vi "mediaIntesecaoCameras_v2.vi"(9 "Lado":enum16{"Esquerdo", "Direito"}(ring) caption="Enum", 10 "Field Geometry In":T3, 11 "Cameras Array":T4[](array[typedef]) {"robots_blue"."height" format="%+4.3f"; "robots_blue"."pixel_y" format="%+4.3f"; "robots_blue"."pixel_x" format="%+4.3f"; "robots_blue"."orientation" format="%+4.3f"; "robots_blue"."y" format="%+4.3f"; "robots_blue"."confidence" format="%4.3f"; "robots_blue"."x" format="%+4.3f"; "robots_yellow"."height" format="%+4.3f"; "robots_yellow"."pixel_y" format="%+4.3f"; "robots_yellow"."pixel_x" format="%+4.3f"; "robots_yellow"."orientation" format="%+4.3f"; "robots_yellow"."y" format="%+4.3f"; "robots_yellow"."confidence" format="%4.3f"; "robots_yellow"."x" format="%+4.3f"}) -> (3 "frame out":T4 {"robots_blue"."height" format="%+4.3f"; "robots_blue"."pixel_y" format="%+4.3f"; "robots_blue"."pixel_x" format="%+4.3f"; "robots_blue"."orientation" format="%+4.3f"; "robots_blue"."y" format="%+4.3f"; "robots_blue"."confidence" format="%4.3f"; "robots_blue"."x" format="%+4.3f"; "robots_yellow"."height" format="%+4.3f"; "robots_yellow"."pixel_y" format="%+4.3f"; "robots_yellow"."pixel_x" format="%+4.3f"; "robots_yellow"."orientation" format="%+4.3f"; "robots_yellow"."y" format="%+4.3f"; "robots_yellow"."confidence" format="%4.3f"; "robots_yellow"."x" format="%+4.3f"})   [LabVIEW 2018]
uses:
  SSL Detection Frame.ctl
  SSL Detection Robot.ctl
  <vilib>/Analysis/Matrix/Datatypes/RealMatrix.ctl
  SSL Detection Ball.ctl
  <vilib>/Analysis/Matrix/NI_Matrix.lvlib
panel:
  in  "Array":T1[](array[typedef])
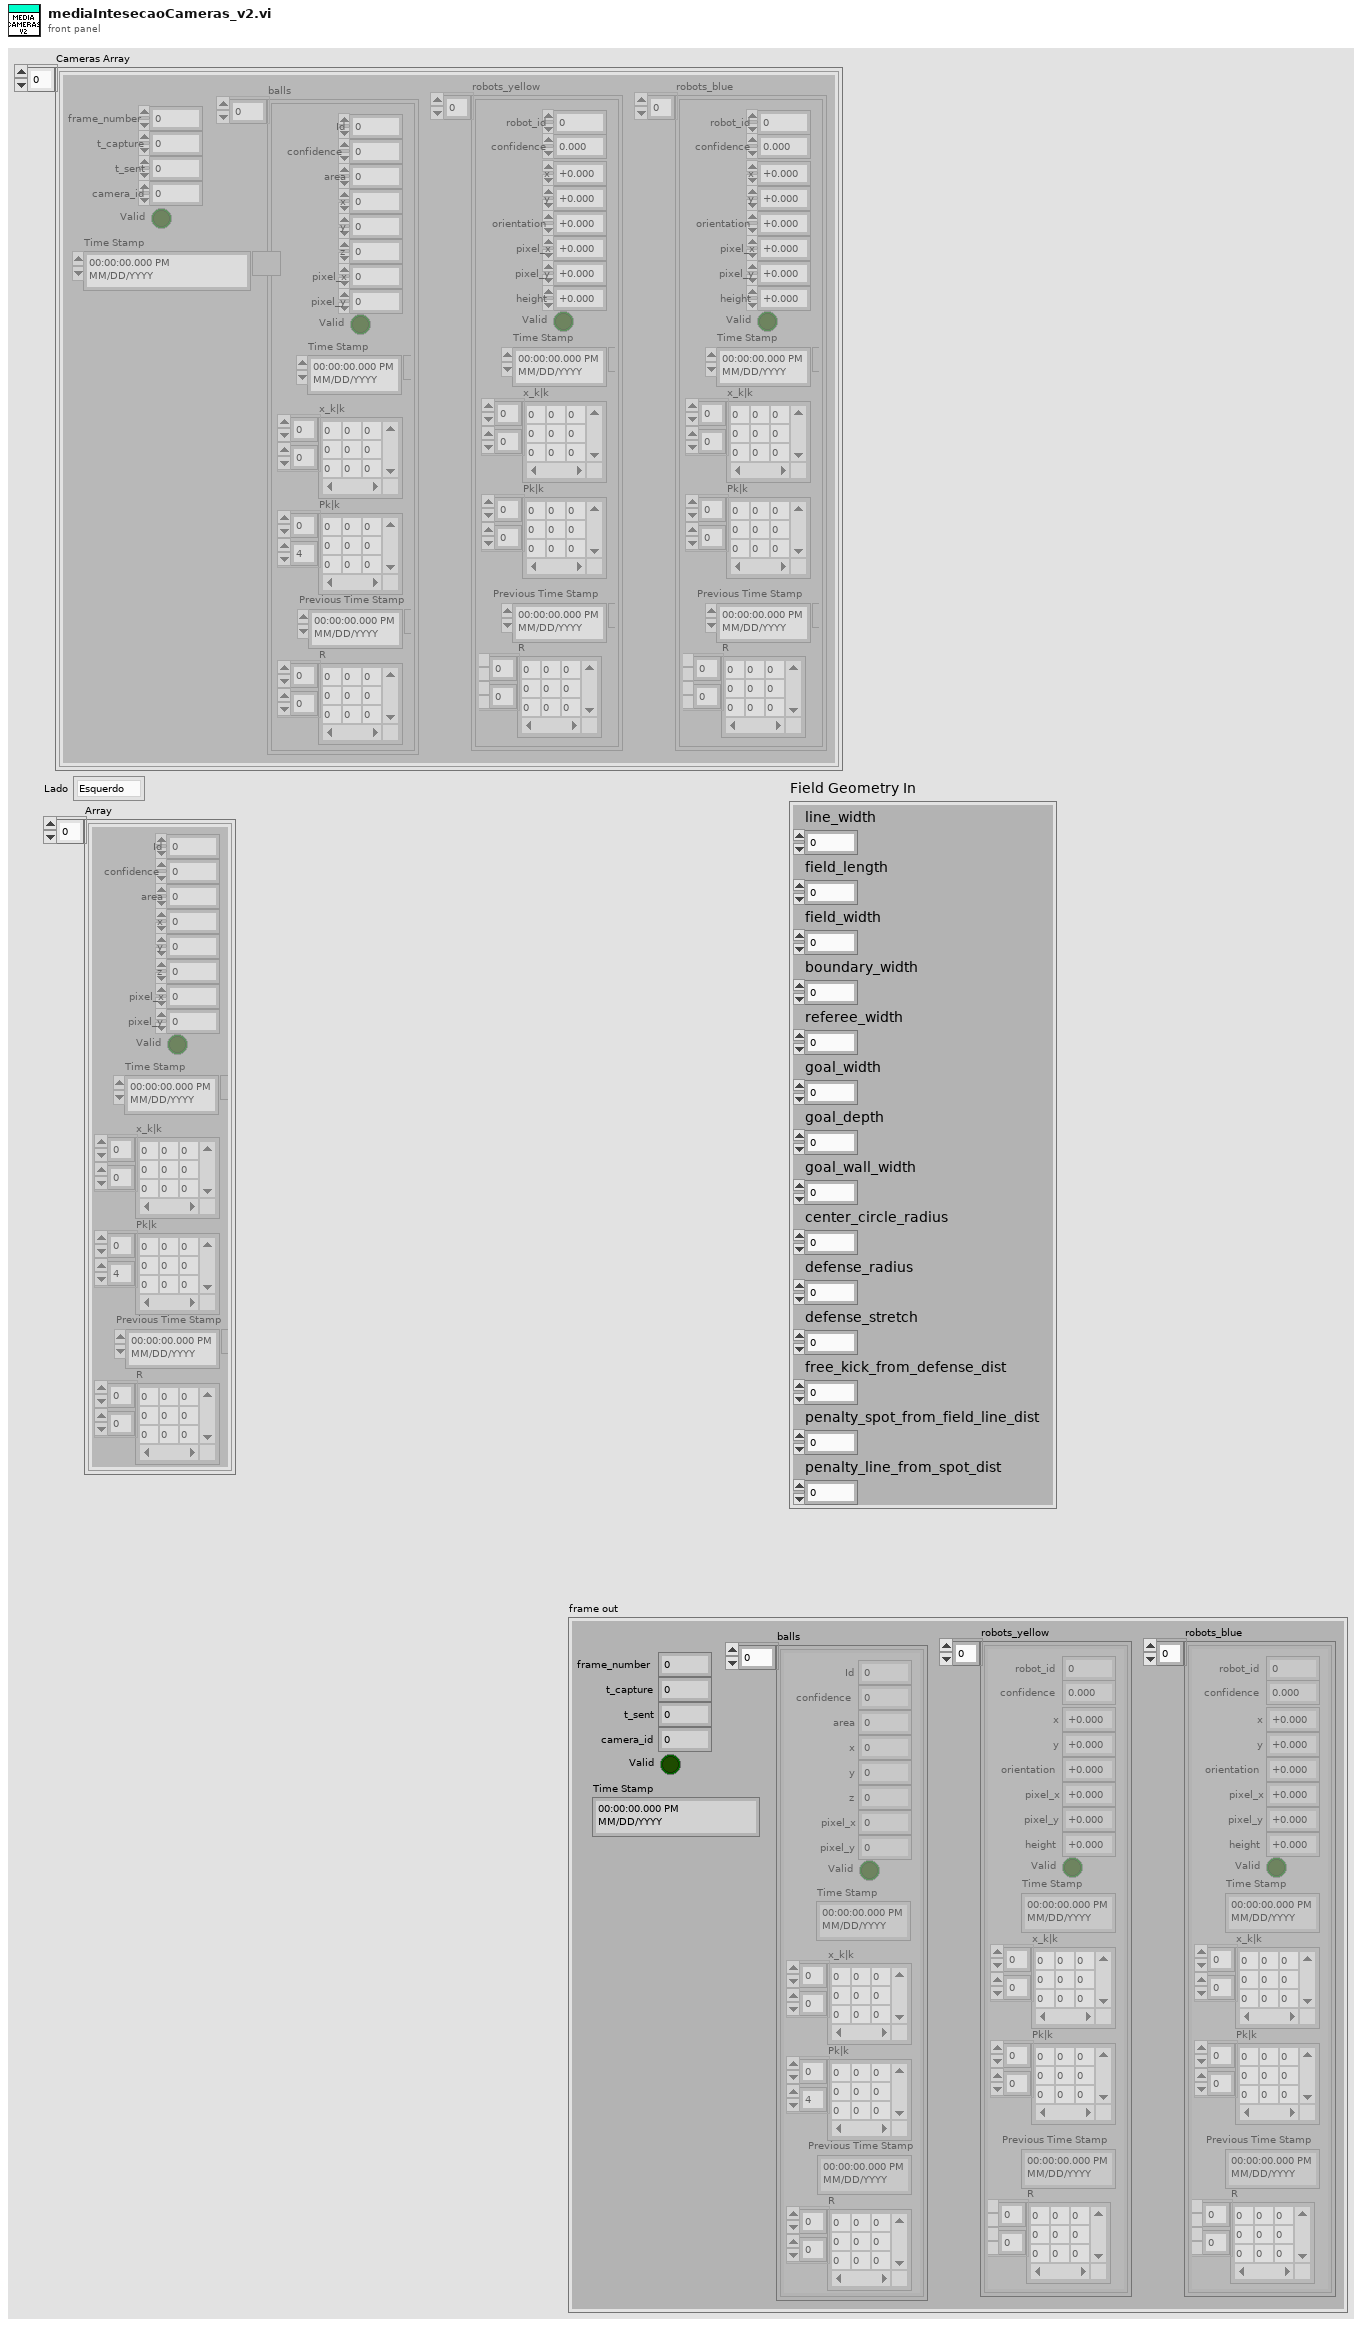
[diagram p1: front panel]
types:
  T1 = typedef "SSL Detection Ball.ctl" = cluster{"x":sgl, "area":u32, "confidence":sgl, "y":sgl, "z":sgl, "pixel_x":sgl, "pixel_y":sgl, "Valid":bool, "Time Stamp":timestamp, "x_k|k":T2, "Pk|k":T2, "Id":u32, "Previous Time Stamp":timestamp, "R":T2}
  T2 = typedef "NI_Matrix.lvlib/RealMatrix.ctl" = dbl[][]
  T3 = cluster{"line_width":u32, "field_length":u32, "field_width":u32, "boundary_width":u32, "referee_width":u32, "goal_width":u32, "goal_depth":u32, "goal_wall_width":u32, "center_circle_radius":u32, "defense_radius":u32, "defense_stretch":u32, "free_kick_from_defense_dist":u32, "penalty_spot_from_field_line_dist":u32, "penalty_line_from_spot_dist":u32}
  T4 = typedef "SSL Detection Frame.ctl" = cluster{"frame_number":u32, "t_capture":dbl, "t_sent":dbl, "camera_id":u32, "robots_yellow":T5[], "robots_blue":T5[], "balls":T1[], "Valid":bool, "Time Stamp":timestamp}
  T5 = typedef "SSL Detection Robot.ctl" = cluster{"x":sgl, "robot_id":u32, "confidence":sgl, "y":sgl, "orientation":sgl, "pixel_x":sgl, "pixel_y":sgl, "height":sgl, "Valid":bool, "Time Stamp":timestamp, "x_k|k":T2, "Pk|k":T2, "Previous Time Stamp":timestamp, "R":T2}
  T6 = cluster{"x":sgl, "y":sgl, "orientation":sgl, "robot_id":u32, "camera_id":u32, "Valid":bool}
  T7 = cluster{"x":sgl, "y":sgl, "camera_id":u32, "Valid":bool}
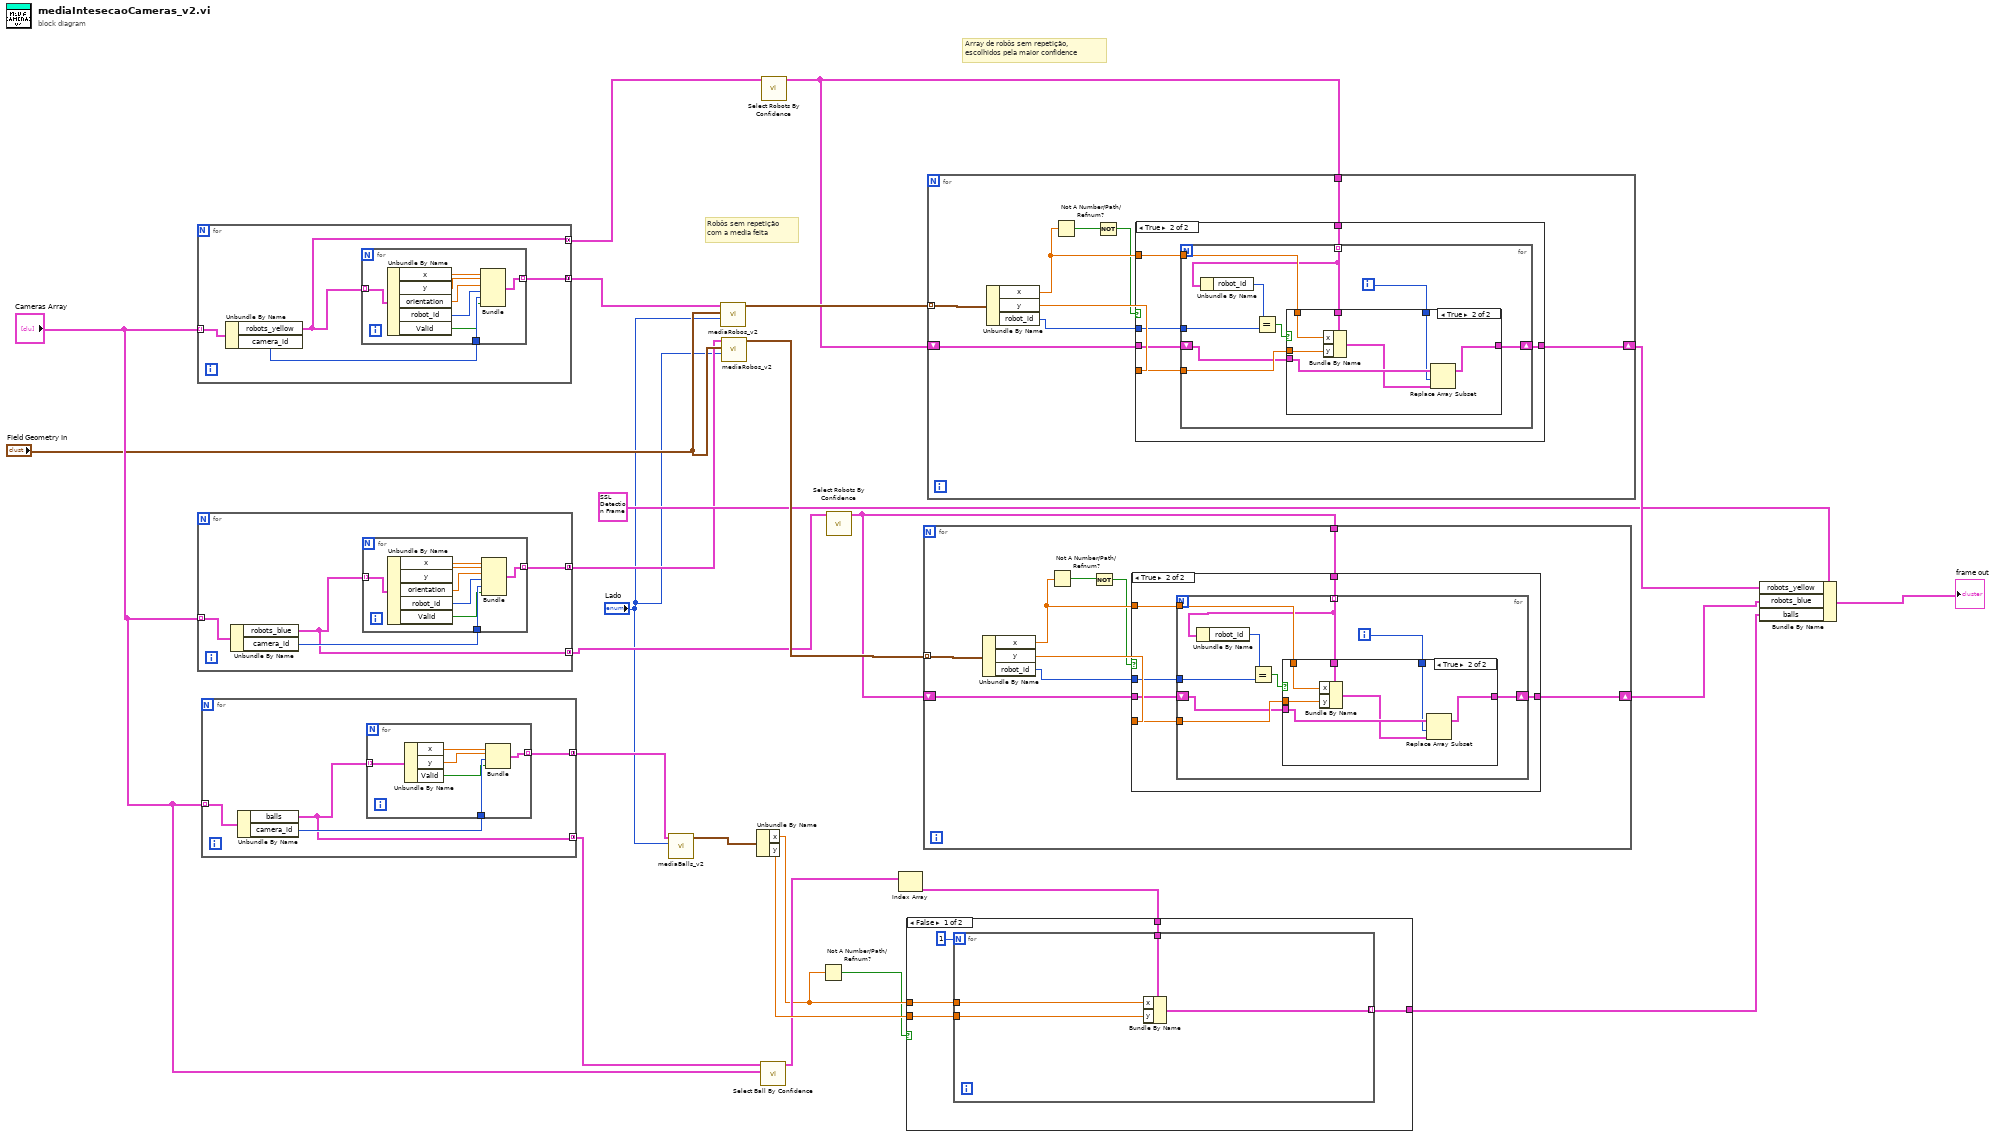
[diagram p0: block diagram]
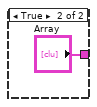
[diagram p2: hidden frame]
diagram:
  # "Robôs sem repetição \ncom a media feita"
  # "Array de robôs sem repetição,\nescolhidos pela maior confidence"
  n1 = for {
    tunnel: "Cameras Array" -> [w28] mode=indexing
    tunnel: [w27] -> w6 mode=concatenating
    tunnel: [w25] -> w20 mode=concatenating
    n2 = Unbundle By Name(w28) -> ("robots_yellow"=w25:T5[], "camera_id"=w26:u32)
    n3 = for {
      tunnel: w25 -> [w36] mode=indexing
      tunnel: [w33] -> w27 mode=indexing
      tunnel: w26 -> [w30]
      n4 = Unbundle By Name(w36) -> ("x"=w35:sgl, "y"=w34:sgl, "orientation"=w32:sgl, "robot_id"=w31:u32, "Valid"=w29:bool)
      n5 = Bundle("x"=w35, "y"=w34, "orientation"=w32, "robot_id"=w31, "camera_id"=w30, "Valid"=w29) -> (w33:T6)  [unwired: 1 in]
    }
  }
  n6 = for {
    tunnel: "Cameras Array" -> [w40] mode=indexing
    tunnel: [w39] -> w5 mode=concatenating
    tunnel: [w37] -> w16 mode=concatenating
    n7 = Unbundle By Name(w40) -> ("robots_blue"=w37:T5[], "camera_id"=w38:u32)
    n8 = for {
      tunnel: w37 -> [w48] mode=indexing
      tunnel: [w45] -> w39 mode=indexing
      tunnel: w38 -> [w42]
      n9 = Unbundle By Name(w48) -> ("x"=w47:sgl, "y"=w46:sgl, "orientation"=w44:sgl, "robot_id"=w43:u32, "Valid"=w41:bool)
      n10 = Bundle("x"=w47, "y"=w46, "orientation"=w44, "robot_id"=w43, "camera_id"=w42, "Valid"=w41) -> (w45:T6)  [unwired: 1 in]
    }
  }
  n11 = for {
    tunnel: "Cameras Array" -> [w52] mode=indexing
    tunnel: [w51] -> w4 mode=concatenating
    tunnel: [w49] -> w13 mode=concatenating
    n12 = Unbundle By Name(w52) -> ("balls"=w49:T1[], "camera_id"=w50:u32)
    n13 = for {
      tunnel: w49 -> [w58] mode=indexing
      tunnel: [w55] -> w51 mode=indexing
      tunnel: w50 -> [w54]
      n14 = Unbundle By Name(w58) -> ("x"=w57:sgl, "y"=w56:sgl, "Valid"=w53:bool)
      n15 = Bundle("x"=w57, "y"=w56, "camera_id"=w54, "Valid"=w53) -> (w55:T7)  [unwired: 1 in]
    }
  }
  n16 = call "mediaBalls_v2.vi"("Lado"="Lado", "Array Ball Pose + CamID"=w4) -> ("Ball out"=w22:cluster{"x":dbl, "y":dbl})  [unwired: 9 in]
  n17 = call "mediaRobos_v2.vi"("Lado"="Lado", "Field Size 2"="Field Geometry In", "Array Robot Pose + CamID"=w6) -> ("Array"=w24:cluster{"x":dbl, "y":dbl, "robot_id":i32}[])  [unwired: 8 in]
  n18 = call "mediaRobos_v2.vi"("Lado"="Lado", "Field Size 2"="Field Geometry In", "Array Robot Pose + CamID"=w5) -> ("Array"=w17:cluster{"x":dbl, "y":dbl, "robot_id":i32}[])  [unwired: 8 in]
  n19 = Unbundle By Name(w22) -> ("x"=w3:dbl, "y"=w21:dbl)
  n20 = call "Select Ball By Confidence.vi"("Array"="Cameras Array", "balls"=w13) -> ("balls out"=w11:T1[])  [unwired: 9 in]
  n21 = call "Select Robots By Confidence.vi"("robots_blue"=w20) -> ("Array"=w19:T5[])  [unwired: 10 in]
  n22 = Not A Number/Path/Refnum?(number/path/refnum=w3) -> (NaN/Path/Refnum?=w2:bool)
  n23 = call "Select Robots By Confidence.vi"("robots_blue"=w16) -> ("Array"=w15:T5[])  [unwired: 10 in]
  n24 = Index Array(array=w11) -> (element=w10:T1)  [unwired: 1 in]
  n25 = case shown="False" w2 {
    tunnel: w21 -> [w63 _]
    tunnel: w10 -> [w62 _]
    tunnel: [w61 "Array"] -> w9
    tunnel: w3 -> [w59 _]
    frame False {
      n26 = for {
        N: 1 -> [_]
        tunnel: w59 -> [w64]
        tunnel: w63 -> [w67]
        tunnel: [w66] -> w61 mode=indexing
        tunnel: w62 -> [w65]
        n27 = Bundle By Name(cluster=w65, "x"=w64, "y"=w67) -> (w66:T1)
      }
    }
    frame True {
    }
  }
  n28 = for {
    tunnel: w17 -> [w77] mode=indexing
    tunnel: w15 -> [w71]
    shift-right: [w75] -> w14
    shift-left: w15 -> [w69]
    n29 = Unbundle By Name(w77) -> ("x"=w74:dbl, "y"=w76:dbl, "robot_id"=w70:i32)
    n30 = Not A Number/Path/Refnum?(number/path/refnum=w74) -> (NaN/Path/Refnum?=w73:bool)
    n31 = Not(x=w73) -> (.not. x?=w72:bool)
    n32 = case shown="True" w72 {
      tunnel: w74 -> [_ w84]
      tunnel: w76 -> [_ w83]
      tunnel: [w78 w82] -> w75
      tunnel: w71 -> [_ w81]
      tunnel: w70 -> [_ w80]
      tunnel: w69 -> [w78 w79]
      frame False {
      }
      frame True {
        n33 = for {
          tunnel: w84 -> [w93]
          tunnel: w83 -> [w92]
          shift-right: [w86] -> w82
          shift-left: w79 -> [w87]
          tunnel: w81 -> [w88] mode=indexing
          tunnel: w80 -> [w90]
          i -> [w85]
          n34 = Unbundle By Name(w88) -> ("robot_id"=w91:u32)
          n35 = Equal?(x=w91, y=w90) -> (x = y?=w89:bool)
          n36 = case shown="True" w89 {
            tunnel: w93 -> [_ w101]
            tunnel: w92 -> [_ w100]
            tunnel: w88 -> [_ w99]
            tunnel: w87 -> [w94 w98]
            tunnel: [w94 w97] -> w86
            tunnel: w85 -> [_ w95]
            frame False {
            }
            frame True {
              n37 = Bundle By Name(cluster=w99, "x"=w101, "y"=w100) -> (w96:T5)
              n38 = Replace Array Subset(array=w98, new element=w96, index=w95) -> (w97:T5[])
            }
          }
        }
      }
    }
  }
  n39 = for {
    tunnel: w24 -> [w110] mode=indexing
    tunnel: w19 -> [w104]
    shift-right: [w108] -> w18
    shift-left: w19 -> [w102]
    n40 = Unbundle By Name(w110) -> ("x"=w107:dbl, "y"=w109:dbl, "robot_id"=w103:i32)
    n41 = Not A Number/Path/Refnum?(number/path/refnum=w107) -> (NaN/Path/Refnum?=w106:bool)
    n42 = Not(x=w106) -> (.not. x?=w105:bool)
    n43 = case shown="True" w105 {
      tunnel: w107 -> [_ w117]
      tunnel: w109 -> [_ w116]
      tunnel: [w111 w115] -> w108
      tunnel: w104 -> [_ w114]
      tunnel: w103 -> [_ w113]
      tunnel: w102 -> [w111 w112]
      frame False {
      }
      frame True {
        n44 = for {
          tunnel: w117 -> [w126]
          tunnel: w116 -> [w125]
          shift-right: [w119] -> w115
          shift-left: w112 -> [w120]
          tunnel: w114 -> [w121] mode=indexing
          tunnel: w113 -> [w123]
          i -> [w118]
          n45 = Unbundle By Name(w121) -> ("robot_id"=w124:u32)
          n46 = Equal?(x=w124, y=w123) -> (x = y?=w122:bool)
          n47 = case shown="True" w122 {
            tunnel: w126 -> [_ w134]
            tunnel: w125 -> [_ w133]
            tunnel: w121 -> [_ w132]
            tunnel: w120 -> [w127 w131]
            tunnel: [w127 w130] -> w119
            tunnel: w118 -> [_ w128]
            frame False {
            }
            frame True {
              n48 = Bundle By Name(cluster=w132, "x"=w134, "y"=w133) -> (w129:T5)
              n49 = Replace Array Subset(array=w131, new element=w129, index=w128) -> (w130:T5[])
            }
          }
        }
      }
    }
  }
  n50 = Bundle By Name(cluster=T4 {"frame_number"=0, "t_capture"=0.0, "t_sent"=0.0, "camera_id"=0, "robots_yellow"=[], "robots_blue"=[], "balls"=[], "Valid"=TRUE, "Time Stamp"=timestamp(0 s since 1904-01-01)} ("Unico frame"), "robots_yellow"=w18, "robots_blue"=w14, "balls"=w9) -> (→"frame out":T4)
